vi "Get Source User Delay.vi"(8 "error in (no error)":errorcluster, 9 "User Delay (1)":i32=1 min=1 max=5 step=1, 10 "Function (0: Volts)":u16(ring) items=["Volts", "Current", "Resistance"], 11 "VISA resource name":refnum<visa-resource-name>) -> (0 "error out":errorcluster, 2 "Delay Time":dbl, 3 "VISA resource name out":refnum<visa-resource-name>)   [LabVIEW 2017, in "Keithley 2450.lvlib"]
doc: "This command gets a source user-defined delay that can be used in the trigger model."
uses:
  Keithley 2450.lvlib
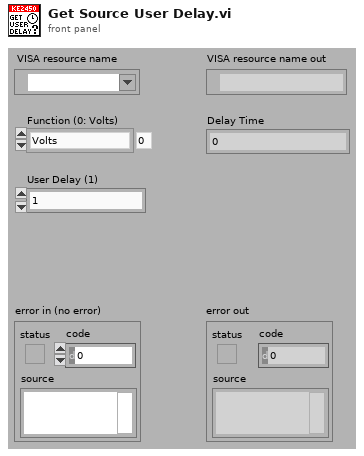
[diagram p1: front panel]
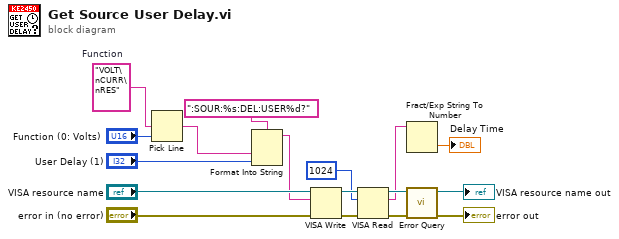
[diagram p0: block diagram]
diagram:
  w11 = "VOLT\nCURR\nRES"  # Function
  n1 = Pick Line(multi-line string=w11, line index="Function (0: Volts)") -> (output string=w9:string)  [unwired: 1 out]
  n2 = Format Into String(format string=":SOUR:%s:DEL:USER%d?", w9, "User Delay (1)") -> (resulting string=w12:string)  [unwired: 2 in, 1 out]
  n3 = VISA Write(VISA resource name="VISA resource name", write buffer=w12, error in (no error)="error in (no error)") -> (VISA resource name out=w7:refnum<visa-resource-name>, error out=w5:errorcluster)  [unwired: 1 out]
  n4 = VISA Read(VISA resource name=w7, byte count=u32 1024, error in (no error)=w5) -> (VISA resource name out=w6:refnum<visa-resource-name>, read buffer=w2:string, error out=w4:errorcluster)  [unwired: 1 out]
  n5 = Fract/Exp String To Number(string=w2) -> (number=→"Delay Time":dbl)  [unwired: 3 in, 1 out]
  n6 = call "Error Query.vi"("error in (no error)"=w4, "VISA resource name"=w6) -> ("error out"=→"error out":errorcluster, "VISA resource name out"=→"VISA resource name out":refnum<visa-resource-name>)  [unwired: 8 out]
